vi "风扇温度.vi"(10 "order":string) -> (0 "temp":string[](array[string]), 3 "fengshan":string[](array[string]))   [LabVIEW 2015]
uses:
  Global/Globalclient.vi
  <vilib>/regexp/Match Regular Expression.xnode
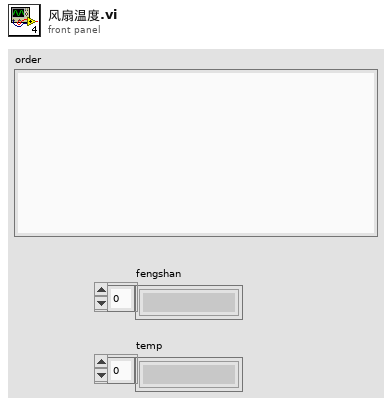
[diagram p1: front panel]
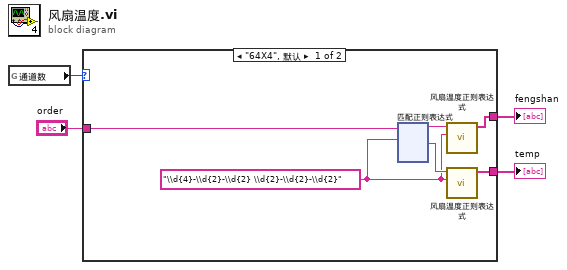
[diagram p0: block diagram]
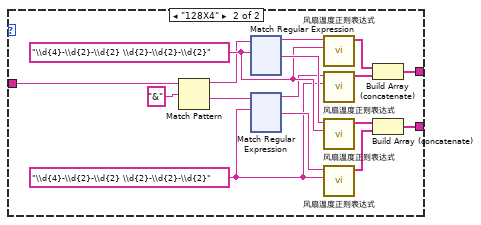
[diagram p2: hidden frame]
diagram:
  n1 = global read "Globalclient.vi" "通道数"() -> (w4:enum16{"64X4", "128X4"})
  n2 = case shown="\"64X4\", 默认" w4 {
    tunnel: [w6 w124] -> w3
    tunnel: [w5 w123] -> w2
    tunnel: "order" -> [w7 w122]
    frame "64X4", Default {
      w8 = "\\d{4}-\\d{2}-\\d{2} \\d{2}-\\d{2}-\\d{2}"
      n3 = xnode "匹配正则表达式"("输入字符串"=w7, "正则表达式"=w8) -> ("匹配之前"=w9:string, "匹配之后"=w10:string)  [unwired: 4 in, 3 out]
      n4 = call "风扇温度正则表达式.vi"("字符串"=w8, "匹配之后"=w9) -> ("temp"=w6:string[])  [unwired: 9 in]
      n5 = call "风扇温度正则表达式.vi"("字符串"=w8, "匹配之后"=w10) -> ("temp"=w5:string[])  [unwired: 9 in]
    }
    frame "128X4" {
      w129 = "\\d{4}-\\d{2}-\\d{2} \\d{2}-\\d{2}-\\d{2}"
      w135 = "\\d{4}-\\d{2}-\\d{2} \\d{2}-\\d{2}-\\d{2}"
      n6 = Match Pattern(string=w122, regular expression="&") -> (before substring=w131:string, after substring=w130:string)  [unwired: 1 in, 2 out]
      n7 = xnode "Match Regular Expression"("输入字符串"=w131, "正则表达式"=w135) -> ("匹配之前"=w136:string, "匹配之后"=w137:string)  [unwired: 4 in, 3 out]
      n8 = xnode "Match Regular Expression"("输入字符串"=w130, "正则表达式"=w129) -> ("匹配之前"=w133:string, "匹配之后"=w132:string)  [unwired: 4 in, 3 out]
      n9 = call "风扇温度正则表达式.vi"("字符串"=w135, "匹配之后"=w136) -> ("temp"=w126:string[])  [unwired: 9 in]
      n10 = call "风扇温度正则表达式.vi"("字符串"=w129, "匹配之后"=w133) -> ("temp"=w125:string[])  [unwired: 9 in]
      n11 = call "风扇温度正则表达式.vi"("字符串"=w135, "匹配之后"=w137) -> ("temp"=w128:string[])  [unwired: 9 in]
      n12 = call "风扇温度正则表达式.vi"("字符串"=w129, "匹配之后"=w132) -> ("temp"=w127:string[])  [unwired: 9 in]
      n13 = Build Array (concatenate)(w126, w125) -> (w124:string[])
      n14 = Build Array (concatenate)(w128, w127) -> (w123:string[])
    }
  }
  "temp" <- w2
  "fengshan" <- w3
